vi "Start Sync.vi"(8 "error in (no error)":errorcluster, 11 "gRPC service in":refnum<class "NI_XNET_CAN_Bus_Monitor_API.lvclass">) -> (0 "error out":errorcluster, 3 "gRPC service out":refnum<class "NI_XNET_CAN_Bus_Monitor_API.lvclass">)   [LabVIEW 2025, in "xnet_can_bus_monitor_api_server.lvlib" / "NI_XNET_CAN_Bus_Monitor_API.lvclass"]
uses:
  NI_XNET_CAN_Bus_Monitor_API.lvclass
  xnet_can_bus_monitor_api_server_do/Types/MainProcess.StateVariables.ctl
  xnet_can_bus_monitor_api_server_do/Types/XNET.InitialSettings.ctl
  RPC Messages/ni_xnet_can_bm_api_ConnectSettings.ctl
  RPC Messages/ni_xnet_can_bm_api_CanMode.ctl
  RPC Messages/ni_xnet_can_bm_api_Termination.ctl
  RPC Messages/ni_xnet_can_bm_api_FdIsoMode.ctl
  RPC Messages/ni_xnet_can_bm_api_FilterInfo.ctl
  RPC Messages/ni_xnet_can_bm_api_DirectionFilter.ctl
  RPC Messages/ni_xnet_can_bm_api_FrameFilter.ctl
  xnet_can_bus_monitor_api_server_do/Types/StreamProcess.Refs.ctl
  xnet_can_bus_monitor_api_server_do/Types/StreamProcess.VIRef.ctl
  NI_XNET_CAN_Bus_Monitor_API.lvclass/NI_XNET_CAN_Bus_Monitor_API.ctl
  xnet_can_bus_monitor_api_server.lvlib
  xnet_can_bus_monitor_api_server_do/xnet_can_bus_monitor_api_server_do.lvlib
  RPC Messages/ni_xnet_can_bm_api_Session.ctl
panel:
  out "Streaming VI status":errorcluster
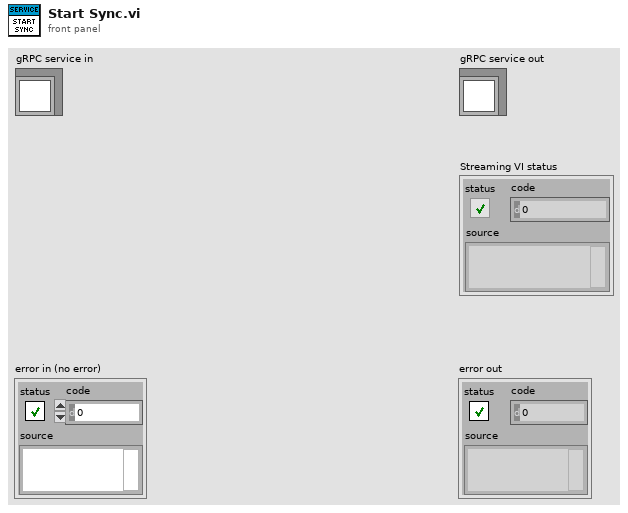
[diagram p1: front panel]
types:
  T1 = typedef "xnet_can_bus_monitor_api_server_do.lvlib/MainProcess.StateVariables.ctl" = cluster{"Settings":T2, "Outgoing.Ref":refnum<k21>, "FilterDVR.Ref":refnum<data-value>, "StreamingVI":T10, "Session":T12}
  T2 = typedef "xnet_can_bus_monitor_api_server_do.lvlib/XNET.InitialSettings.ctl" = cluster{"Name":string, "Port Settings":T3, "Default Filter":T7}
  T3 = typedef "xnet_can_bus_monitor_api_server.lvlib/ni_xnet_can_bm_api_ConnectSettings.ctl" = cluster{"port":string, "can_mode":T4, "termination":T5, "baud_rate":u64, "fd_baud_rate":u64, "fd_iso_mode":T6}
  T4 = typedef "xnet_can_bus_monitor_api_server.lvlib/ni_xnet_can_bm_api_CanMode.ctl" = enum32{"CAN_2", "CAN_FD", "CAN_FD_BRS"}
  T5 = typedef "xnet_can_bus_monitor_api_server.lvlib/ni_xnet_can_bm_api_Termination.ctl" = enum32{"Term_Off", "Term_On"}
  T6 = typedef "xnet_can_bus_monitor_api_server.lvlib/ni_xnet_can_bm_api_FdIsoMode.ctl" = enum32{"ISO", "Non_ISO", "ISO_Legacy"}
  T7 = typedef "xnet_can_bus_monitor_api_server.lvlib/ni_xnet_can_bm_api_FilterInfo.ctl" = cluster{"filter_ids":u32[], "direction_filter":T8, "frame_filter":T9}
  T8 = typedef "xnet_can_bus_monitor_api_server.lvlib/ni_xnet_can_bm_api_DirectionFilter.ctl" = enum32{"TX_RX", "RX", "TX"}
  T9 = typedef "xnet_can_bus_monitor_api_server.lvlib/ni_xnet_can_bm_api_FrameFilter.ctl" = enum32{"CAN_Data", "CAN_Remote", "CAN_Bus_Error", "CAN_2_Data", "CAN_FD_Data", "CAN_FD_BRS_Data", "J1939_Data", "Delay", "Log_Trigger", "Start_Trigger", "All"}
  T10 = typedef "xnet_can_bus_monitor_api_server_do.lvlib/StreamProcess.Refs.ctl" = cluster{"Ref":T11, "Stop":refnum<notifier>, "Error":refnum<notifier>}
  T11 = typedef "xnet_can_bus_monitor_api_server_do.lvlib/StreamProcess.VIRef.ctl" = refnum<vi>
  T12 = typedef "xnet_can_bus_monitor_api_server.lvlib/ni_xnet_can_bm_api_Session.ctl" = cluster{"name":string, "session_uid":string}
  T13 = typedef "xnet_can_bus_monitor_api_server.lvlib/NI_XNET_CAN_Bus_Monitor_API.lvclass/Server Internal UEs.ctl" = cluster{"NI_XNET_CAN_Bus_Monitor_API PassThru Internal UE":refnum<user-event>, "NI_XNET_CAN_Bus_Monitor_API GetStreamingFilter Internal UE":refnum<user-event>, "NI_XNET_CAN_Bus_Monitor_API SetStreamingFilter Internal UE":refnum<user-event>, "NI_XNET_CAN_Bus_Monitor_API ResetStreamingFilter Internal UE":refnum<user-event>, "NI_XNET_CAN_Bus_Monitor_API InitializeSettings Internal UE":refnum<user-event>, "NI_XNET_CAN_Bus_Monitor_API StopProcess Internal UE":refnum<user-event>, "NI_XNET_CAN_Bus_Monitor_API StreamBus Internal UE":refnum<user-event>}
  T14 = typedef "xnet_can_bus_monitor_api_server.lvlib/NI_XNET_CAN_Bus_Monitor_API.lvclass/Server gRPC UEs.ctl" = cluster{"NI_XNET_CAN_Bus_Monitor_API PassThru gRPC UE":refnum<user-event>, "NI_XNET_CAN_Bus_Monitor_API GetStreamingFilter gRPC UE":refnum<user-event>, "NI_XNET_CAN_Bus_Monitor_API SetStreamingFilter gRPC UE":refnum<user-event>, "NI_XNET_CAN_Bus_Monitor_API ResetStreamingFilter gRPC UE":refnum<user-event>, "NI_XNET_CAN_Bus_Monitor_API InitializeSettings gRPC UE":refnum<user-event>, "NI_XNET_CAN_Bus_Monitor_API StopProcess gRPC UE":refnum<user-event>, "NI_XNET_CAN_Bus_Monitor_API StreamBus gRPC UE":refnum<user-event>}
  T15 = typedef "grpc-lvsupport-release.lvlib/grpcId.ctl" = u64
  T16 = typedef "xnet_can_bus_monitor_api_server.lvlib/ni_xnet_can_bm_api_InitializeSettingsRequest.ctl" = cluster{"name":string, "connect_settings":T3, "default_filter_ids":u32[]}
  T17 = typedef "xnet_can_bus_monitor_api_server.lvlib/ni_xnet_can_bm_api_InitializeSettingsReply.ctl" = cluster{"session":T12, "error":T18}
  T18 = typedef "xnet_can_bus_monitor_api_server.lvlib/ni_xnet_can_bm_api_ErrorInfo.ctl" = errorcluster
  T19 = typedef "xnet_can_bus_monitor_api_server.lvlib/ni_xnet_can_bm_api_PassThruRequest.ctl" = cluster{"session":T12, "frame":T20}
  T20 = typedef "xnet_can_bus_monitor_api_server.lvlib/ni_xnet_can_bm_api_Frame.ctl" = cluster{"timestamp":dbl, "payload":u8[], "identifier":u32, "frame_type":u32, "extended":bool, "echo":bool}
  T21 = typedef "xnet_can_bus_monitor_api_server.lvlib/ni_xnet_can_bm_api_PassThruReply.ctl" = cluster{"error":T18}
  T22 = typedef "xnet_can_bus_monitor_api_server.lvlib/ni_xnet_can_bm_api_GetStreamingFilterRequest.ctl" = cluster{"session":T12}
  T23 = typedef "xnet_can_bus_monitor_api_server.lvlib/ni_xnet_can_bm_api_GetStreamingFilterReply.ctl" = cluster{"filter_info":T7, "error":T18}
  T24 = typedef "xnet_can_bus_monitor_api_server.lvlib/ni_xnet_can_bm_api_SetStreamingFilterRequest.ctl" = cluster{"session":T12, "filter_info":T7}
  T25 = typedef "xnet_can_bus_monitor_api_server.lvlib/ni_xnet_can_bm_api_SetStreamingFilterReply.ctl" = cluster{"error":T18}
  T26 = typedef "xnet_can_bus_monitor_api_server.lvlib/ni_xnet_can_bm_api_ResetStreamingFilterRequest.ctl" = cluster{"session":T12}
  T27 = typedef "xnet_can_bus_monitor_api_server.lvlib/ni_xnet_can_bm_api_ResetStreamingFilterReply.ctl" = cluster{"filter_info":T7, "error":T18}
  T28 = typedef "xnet_can_bus_monitor_api_server.lvlib/ni_xnet_can_bm_api_StopProcessRequest.ctl" = cluster{"session":T12}
  T29 = typedef "xnet_can_bus_monitor_api_server.lvlib/ni_xnet_can_bm_api_StopProcessReply.ctl" = cluster{"stopped":bool, "error":T18}
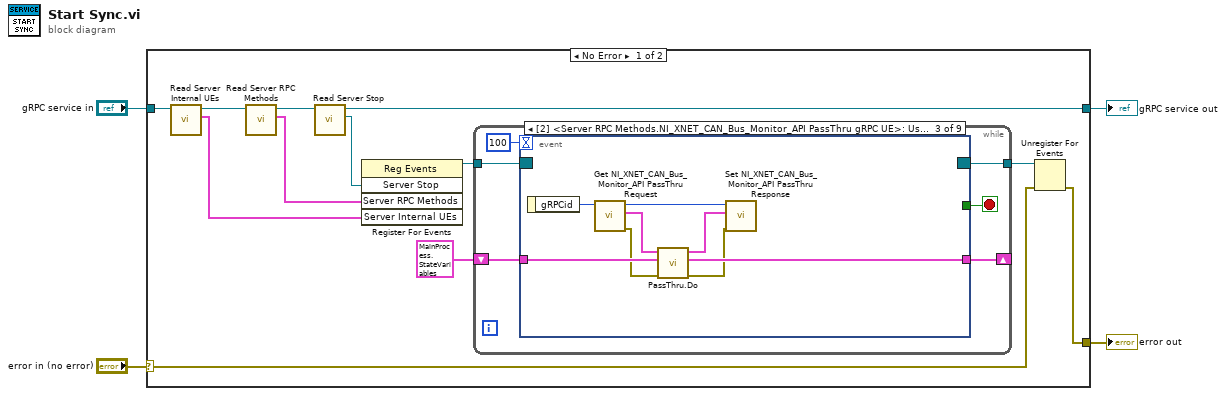
[diagram p0: block diagram]
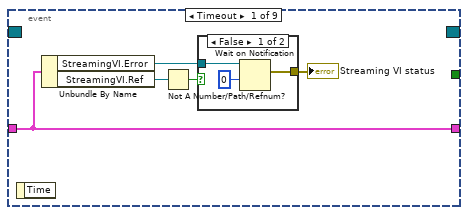
[diagram p2: hidden frame]
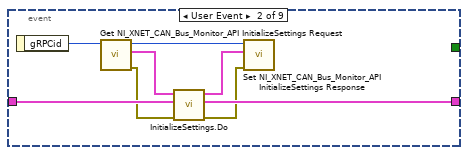
[diagram p4: hidden frame]
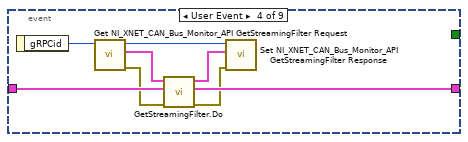
[diagram p5: hidden frame]
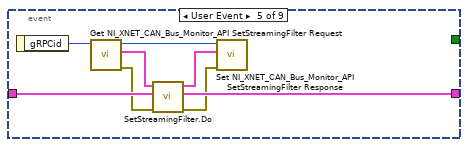
[diagram p6: hidden frame]
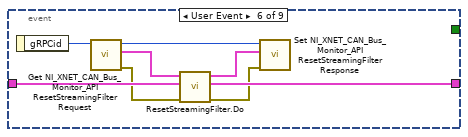
[diagram p7: hidden frame]
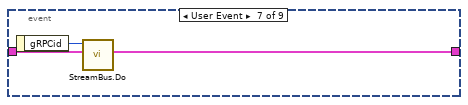
[diagram p8: hidden frame]
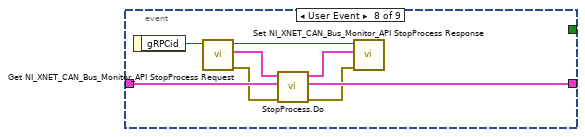
[diagram p9: hidden frame]
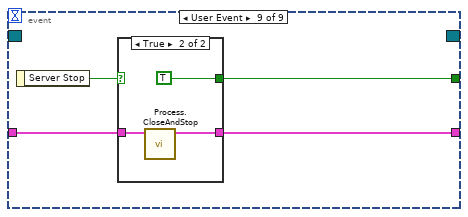
[diagram p10: hidden frame]
diagram:
  n1 = case shown="No Error" "error in (no error)" {
    selector: "error in (no error)" -> [w10 w92]
    tunnel: [w9 w92] -> w3
    tunnel: [w7 w91] -> w1
    tunnel: "gRPC service in" -> [w16 w91]
    frame No Error {
      n2 = call "Read Server Internal UEs.vi"("gRPC service in"=w16) -> ("Server Internal UEs"=w14:T13, "gRPC service out"=w15:refnum<class "NI_XNET_CAN_Bus_Monitor_API.lvclass">)  [unwired: 8 in, 1 out]
      n3 = call "Read Server RPC Methods.vi"("gRPC service in"=w15) -> ("Server RPC Methods"=w8:T14, "gRPC service out"=w13:refnum<class "NI_XNET_CAN_Bus_Monitor_API.lvclass">)  [unwired: 8 in, 1 out]
      n4 = call-dynamic "Read Server Stop.vi"("gRPC service in"=w13) -> ("Server Stop"=w6:refnum<user-event>, "gRPC service out"=w7:refnum<class "NI_XNET_CAN_Bus_Monitor_API.lvclass">)  [unwired: 8 in, 1 out]
      n5 = register-events(w6, w8, w14) -> (reference out=w12:refnum<event-registration>)  [unwired: 2 in, 1 out]
      n6 = while {
        tunnel: w12 -> [w22]
        tunnel: [w20] -> w11
        shift-right: [w18] -> _
        shift-left: T1 {"Settings"={"Name"="", "Port Settings"={"port"="", "can_mode"=enum."CAN_2", "termination"=enum."Term_Off", "baud_rate"=0, "fd_baud_rate"=0, "fd_iso_mode"=enum."ISO"}, "Default Filter"={"filter_ids"=[], "direction_filter"=enum."TX_RX", "frame_filter"=enum."CAN_Data"}}, "Outgoing.Ref"="", "FilterDVR.Ref"=refnum, "StreamingVI"={"Ref"=refnum, "Stop"=refnum, "Error"=refnum}, "Session"={"name"="", "session_uid"=""}} ("cluster") -> [w17]
        stop <- w21 stop-if-true
        n7 = event "RPC Methods Event Structure" shown="[2] <Server RPC Methods.NI_XNET_CAN_Bus_Monitor_API PassThru gRPC UE>: User Event" {
          selector: w22 -> [_ _ _ _ _ _ _ _ _]
          dyn-events: [_ _ _ _ _ _ _ _ _] -> w20
          timeout: 100 -> [_ _ _ _ _ _ _ _ _]
          tunnel: [_ _ _ _ _ _ _ _ w85] -> w21
          tunnel: [w27 w34 w42 w51 w58 w66 w71 w81 w82] -> w18
          tunnel: w17 -> [w27 w33 w41 w50 w57 w65 w72 w80 w83]
          event Timeout {
            n8 = event-data() -> ()  [unwired: 1 in, 1 out]
            n9 = Unbundle By Name(w27) -> ("StreamingVI.Error"=w24:refnum<notifier>, "StreamingVI.Ref"=w26:T11)
            n10 = Not A Number/Path/Refnum?(number/path/refnum=w26) -> (NaN/Path/Refnum?=w25:bool)
            n11 = case shown="False" w25 {
              tunnel: w24 -> [w30 _]
              tunnel: [w28 _] -> w23
              frame False {
                n12 = Wait on Notification(notifier=w30, timeout in ms (-1)=0) -> (notification=w28:errorcluster)  [unwired: 2 in, 3 out]
              }
              frame True {
              }
            }
            "Streaming VI status" <- w23
          }
          event User Event {
            n13 = event-data() -> ("gRPCid"=w38:T15)  [unwired: 1 in]
            n14 = call "Get NI_XNET_CAN_Bus_Monitor_API InitializeSettings Request.vi"("gRPCid"=w38) -> ("error out"=w32:errorcluster, "Message Data"=w36:T16, "gRPCid out"=w37:T15)  [unwired: 8 in]
            n15 = call "InitializeSettings.Do.vi"("error in (no error)"=w32, "State Variables"=w33, "gRPC Request"=w36) -> ("error out"=w31:errorcluster, "State Variables out"=w34:T1, "gRPC Response"=w35:T17)  [unwired: 6 in]
            n16 = call "Set NI_XNET_CAN_Bus_Monitor_API InitializeSettings Response.vi"("error in (no error)"=w31, "Message Data"=w35, "gRPCid in"=w37) -> ()  [unwired: 8 in, 1 out]
          }
          event User Event {
            n17 = event-data() -> ("gRPCid"=w46:T15)  [unwired: 1 in]
            n18 = call "Get NI_XNET_CAN_Bus_Monitor_API PassThru Request.vi"("gRPCid"=w46) -> ("error out"=w40:errorcluster, "Message Data"=w45:T19, "gRPCid out"=w44:T15)  [unwired: 8 in]
            n19 = call "PassThru.Do.vi"("error in (no error)"=w40, "State Variables"=w41, "gRPC Request"=w45) -> ("error out"=w39:errorcluster, "State Variables out"=w42:T1, "gRPC Response"=w43:T21)  [unwired: 6 in]
            n20 = call "Set NI_XNET_CAN_Bus_Monitor_API PassThru Response.vi"("error in (no error)"=w39, "Message Data"=w43, "gRPCid in"=w44) -> ()  [unwired: 8 in, 1 out]
          }
          event User Event {
            n21 = event-data() -> ("gRPCid"=w52:T15)  [unwired: 1 in]
            n22 = call "Get NI_XNET_CAN_Bus_Monitor_API GetStreamingFilter Request.vi"("gRPCid"=w52) -> ("error out"=w48:errorcluster, "Message Data"=w49:T22, "gRPCid out"=w54:T15)  [unwired: 8 in]
            n23 = call "GetStreamingFilter.Do.vi"("error in (no error)"=w48, "State Variables"=w50, "gRPC Request"=w49) -> ("error out"=w47:errorcluster, "State Variables out"=w51:T1, "gRPC Response"=w53:T23)  [unwired: 6 in]
            n24 = call "Set NI_XNET_CAN_Bus_Monitor_API GetStreamingFilter Response.vi"("error in (no error)"=w47, "Message Data"=w53, "gRPCid in"=w54) -> ()  [unwired: 8 in, 1 out]
          }
          event User Event {
            n25 = event-data() -> ("gRPCid"=w62:T15)  [unwired: 1 in]
            n26 = call "Get NI_XNET_CAN_Bus_Monitor_API SetStreamingFilter Request.vi"("gRPCid"=w62) -> ("error out"=w56:errorcluster, "Message Data"=w60:T24, "gRPCid out"=w61:T15)  [unwired: 8 in]
            n27 = call "SetStreamingFilter.Do.vi"("error in (no error)"=w56, "State Variables"=w57, "gRPC Request"=w60) -> ("error out"=w55:errorcluster, "State Variables out"=w58:T1, "gRPC Response"=w59:T25)  [unwired: 6 in]
            n28 = call "Set NI_XNET_CAN_Bus_Monitor_API SetStreamingFilter Response.vi"("error in (no error)"=w55, "Message Data"=w59, "gRPCid in"=w61) -> ()  [unwired: 8 in, 1 out]
          }
          event User Event {
            n29 = event-data() -> ("gRPCid"=w70:T15)  [unwired: 1 in]
            n30 = call "Get NI_XNET_CAN_Bus_Monitor_API ResetStreamingFilter Request.vi"("gRPCid"=w70) -> ("error out"=w64:errorcluster, "Message Data"=w67:T26, "gRPCid out"=w69:T15)  [unwired: 8 in]
            n31 = call "ResetStreamingFilter.Do.vi"("error in (no error)"=w64, "State Variables"=w65, "gRPC Request"=w67) -> ("error out"=w63:errorcluster, "State Variables out"=w66:T1, "gRPC Response"=w68:T27)  [unwired: 6 in]
            n32 = call "Set NI_XNET_CAN_Bus_Monitor_API ResetStreamingFilter Response.vi"("error in (no error)"=w63, "Message Data"=w68, "gRPCid in"=w69) -> ()  [unwired: 8 in, 1 out]
          }
          event User Event {
            n33 = event-data() -> ("gRPCid"=w73:T15)  [unwired: 1 in]
            n34 = call "StreamBus.Do.vi"("State Variables"=w72, "gRPCid"=w73) -> ("State Variables out"=w71:T1)  [unwired: 9 in]
          }
          event User Event {
            n35 = event-data() -> ("gRPCid"=w79:T15)  [unwired: 1 in]
            n36 = call "Get NI_XNET_CAN_Bus_Monitor_API StopProcess Request.vi"("gRPCid"=w79) -> ("error out"=w75:errorcluster, "Message Data"=w78:T28, "gRPCid out"=w77:T15)  [unwired: 8 in]
            n37 = call "StopProcess.Do.vi"("error in"=w75, "State Variables"=w80, "gRPC Request"=w78) -> ("error out"=w74:errorcluster, "State Variables out"=w81:T1, "gRPC Response"=w76:T29)  [unwired: 6 in]
            n38 = call "Set NI_XNET_CAN_Bus_Monitor_API StopProcess Response.vi"("error in (no error)"=w74, "Message Data"=w76, "gRPCid in"=w77) -> ()  [unwired: 8 in, 1 out]
          }
          event User Event {
            n39 = event-data() -> ("Server Stop"=w84:bool)  [unwired: 1 in]
            n40 = case shown="True" w84 {
              selector: w84 -> [w87 _]
              tunnel: [w87 TRUE] -> w85
              tunnel: w83 -> [w86 w89]
              tunnel: [w86 w88] -> w82
              frame False {
              }
              frame True {
                n41 = call "Process.CloseAndStop.vi"("State Variables"=w89) -> ("State Variables"=w88:T1)  [unwired: 9 in, 1 out]
              }
            }
          }
        }
      }
      n42 = Unregister For Events(event registration refnum=w11, error in=w10) -> (error out=w9:errorcluster)
    }
    frame Error {
    }
  }
  "error out" <- w3
  "gRPC service out" <- w1
